vi "Get Desired Size.vi"(8 "error in (no error)":errorcluster, 11 "2DArrayPanel2 in":refnum<class "2DArrayPanel2.lvclass">) -> (0 "error out":errorcluster, 2 "Desired Size":T1, 3 "2DArrayPanel2 out":refnum<class "2DArrayPanel2.lvclass">)   [LabVIEW 2020, in "2D Array Example.lvlib" / "2DArrayPanel2.lvclass"]
uses:
  2DArrayPanel2.lvclass
  OOPanel/Desired Size.ctl
  OOPanel/OOPanel.lvlib
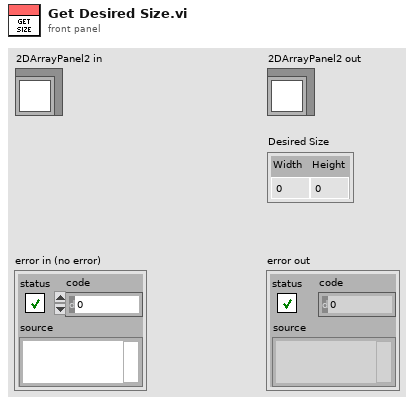
[diagram p1: front panel]
types:
  T1 = typedef "OOPanel.lvlib/Desired Size.ctl" = cluster{"Width":u32, "Height":u32}
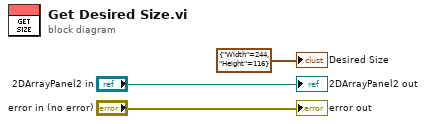
[diagram p0: block diagram]
diagram:
  "error out" <- "error in (no error)"
  "2DArrayPanel2 out" <- "2DArrayPanel2 in"
  "Desired Size" <- T1 {"Width"=244, "Height"=116} ("Desired Size")
